vi "TDMS.FindResult.vi"(11 "Property in":string) -> (1 "Property Text":string, 2 "Result":bool, 3 "Property out":string)   [LabVIEW 2015, in "NIAnalysis.lvlib"]
uses:
  NIAnalysis.lvlib
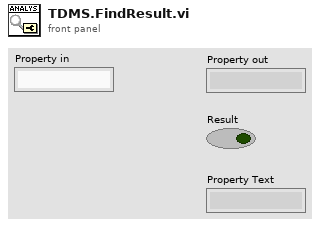
[diagram p1: front panel]
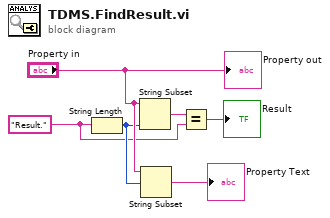
[diagram p0: block diagram]
diagram:
  w1 = "Result." ("string")
  n1 = String Length(string=w1) -> (length=w3:i32)
  n2 = String Subset(string="Property in", length (rest)=w3) -> (substring=w5:string)  [unwired: 1 in]
  n3 = String Subset(string="Property in", offset (0)=w3) -> (substring=→"Property Text":string)  [unwired: 1 in]
  n4 = Equal?(x=w5, y=w1) -> (x = y?=→"Result":bool)
  "Property out" <- "Property in"
